vi "SetGearManipulatorAngle.vi"(10 "Gear Manipulator Angle":dbl, 11 "Gear Manipulator in":refnum<class "Gear Manipulator.lvclass">) -> (3 "Gear Manipulator out":refnum<class "Gear Manipulator.lvclass">)   [LabVIEW 2016, in "Gear Manipulator.lvclass"]
uses:
  Gear Manipulator.lvclass
  Gear Manipulator.lvclass/Gear Manipulator.ctl
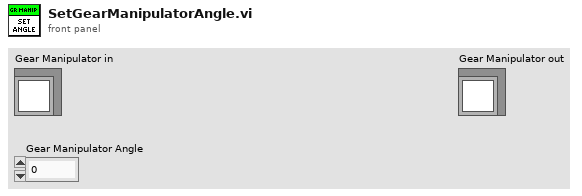
[diagram p1: front panel]
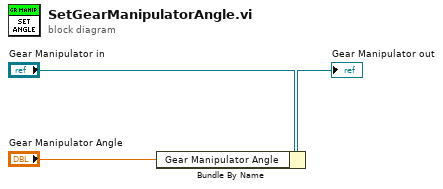
[diagram p0: block diagram]
diagram:
  n1 = Bundle By Name(cluster="Gear Manipulator in", "Gear Manipulator Angle"="Gear Manipulator Angle") -> (→"Gear Manipulator out":refnum<class "Gear Manipulator.lvclass">)
